vi "test.vi"() -> ()   [LabVIEW 2009]
uses:
  ControlProject/PWM/PWM_Name.ctl
  Camera.lvlib
  ControlProject/FPGA.lvlib
  ControlProject/PWM.lvlib
panel:
  in  "High (uSec) 2":u32
  in  "High (uSec)":u32
  out "Image Out":T1(plugin-control)
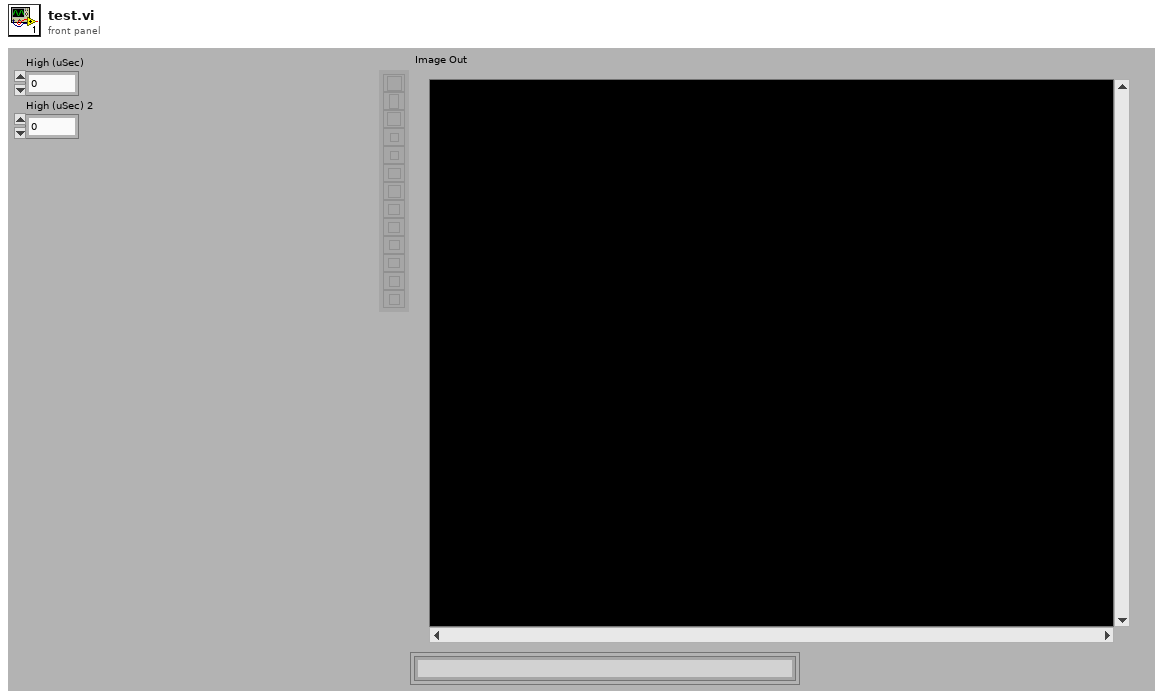
[diagram p1: front panel]
types:
  T1 = typedef "IMAQ Image.ctl" = refnum<image>
  T2 = typedef "PWM.lvlib/PWM_Name.ctl" = u16
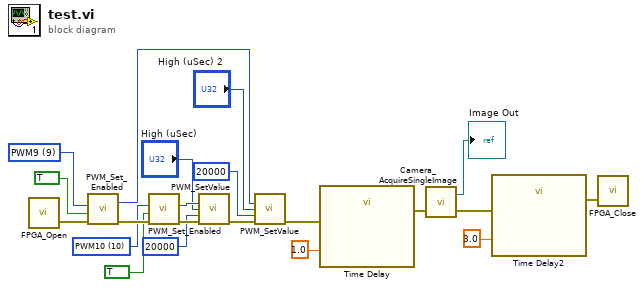
[diagram p0: block diagram]
diagram:
  w12 = T2 9 items=["Invalid"=0, "PWM1"=1, "PWM2"=2, "PWM9"=9, "PWM10"=10] ("PWM_in")
  w13 = T2 10 items=["Invalid"=0, "PWM1"=1, "PWM2"=2, "PWM9"=9, "PWM10"=10] ("PWM_in")
  n1 = call "FPGA_Open.vi"() -> ("error out"=w15:errorcluster)  [unwired: 3 in]
  n2 = call "PWM_Set_Enabled.vi"("error in"=w15, "Enable"=TRUE, "PWM_in"=w12) -> ("error out"=w14:errorcluster, "PWM_out"=w6:T2)  [unwired: 7 in]
  n3 = call "PWM_Set_Enabled.vi"("error in"=w14, "Enable"=TRUE, "PWM_in"=w13) -> ("error out"=w9:errorcluster, "PWM_out"=w8:T2)  [unwired: 7 in]
  n4 = call "PWM_SetValue.vi"("PWM"=w8, "High (uSec)"="High (uSec)", "Period (uSec)"=u32 20000, "error in"=w9) -> ("error out"=w7:errorcluster)  [unwired: 11 in]
  n5 = call "PWM_SetValue.vi"("PWM"=w6, "High (uSec)"="High (uSec) 2", "Period (uSec)"=u32 20000, "error in"=w7) -> ("error out"=w1:errorcluster)  [unwired: 11 in]
  n6 = call "Time Delay"("error in (no error)"=w1, "Delay Time (s)"=1.0) -> ("error out"=w20:errorcluster)  [unwired: 9 in]
  n7 = call "Camera_AcquireSingleImage.vi"("error in"=w20) -> ("error out"=w17:errorcluster, "Image Out"=→"Image Out":T1)  [unwired: 1 in]
  n8 = call "Time Delay2"("error in (no error)"=w17, "Delay Time (s)"=3.0) -> ("error out"=w16:errorcluster)  [unwired: 9 in]
  n9 = call "FPGA_Close.vi"("error in (no error)"=w16) -> ()  [unwired: 2 in, 1 out]
